vi "File Extension.vi"(8 "error in (no error)":errorcluster, 11 "GPack File in":refnum<class "GPack File.lvclass">) -> (0 "error out":errorcluster, 2 "File Extension":string)   [LabVIEW 2020, in "GPack.lvlib" / "GPack File.lvclass"]
uses:
  GPack File.lvclass
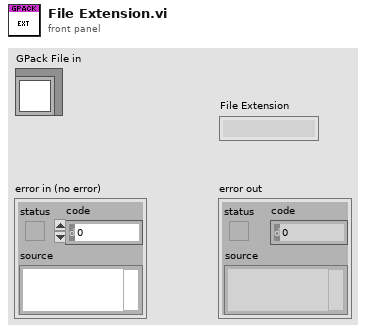
[diagram p1: front panel]
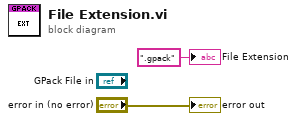
[diagram p0: block diagram]
diagram:
  "error out" <- "error in (no error)"
  "File Extension" <- ".gpack" ("File Extension")
